vi "SVFA Unit Conversion (Colormap).vi"(0 "colormap":T9, 1 "desired scaling":T2 {"dB reference (0: no change)" format="%.2f"}, 2 "spectral density desired":T1(ring), 4 "spectrum info in":T3={"channel name"="", "description"="", "x-axis units"=0, "spectral info"={"spectrum type"=enum."Power [Magnitude^2]", "linear/dB"=enum."linear", "window"=0, "window size"=0, "FFT size"=0}, "engineering units"=0, "custom label"="", "dB reference [EU]"=0.0, "peak units"=enum."rms", "weighting filter"=0, "spectral density?"=FALSE, "unit label"="", "spectrum skewed?"=FALSE, "complimentary spectrum units"=enum."none"} {"x-axis units" items=["Time (s)"=0, "Frequency-CB (Hz)"=1, "Frequency-CPB (Hz)"=1248, "Frequency-Arbitrary (Hz)"=2357, "Quefrency (s)"=2, "Revolutions (rev)"=3, "Order"=4, "Speed (RPM)"=11, "Speed (rad/s)"=21, "Index"=65535]; "weighting filter" items=["Linear", "A-weighting", "B-weighting", "C-weighting", "ITU-R 468-4", "Dolby", "CCITT", "C-message", "Wb", "Wc", "Wd", "We", "Wf", "Wh", "Wj", "Wk", "Wm", "AES17 20 kHz lowpass", "AES17 40 kHz lowpass", "AES17 20 kHz highpass", "AES17 40 kHz highpass"]; "dB reference [EU]" format="%.2f"; "engineering units" items=["custom..."=0, "V"=1, "A"=21, "C"=30, "pC"=31, "s"=32, "-"=29, "Pa"=2, "N"=20, "g"=3, "m/s^2"=4, "m/s"=5, "m"=6, "mm/s"=12, "mm"=13, "micron/s"=14, "micron"=15, "in/s^2"=7, "in/s"=8, "in"=9, "mil/s"=10, "mil"=11, "rad/s^2"=16, "rad/s"=17, "rad"=18, "deg/s^2"=26, "deg/s"=27, "deg"=28, "RPM"=22, "cycle/s^2"=23, "Hz"=24, "cycle"=25, "strain"=19]; "spectral info"."window" items=["None "=0, "Hanning"=1, "Hamming"=2, "Blackman-Harris"=3, "Exact Blackman"=4, "Blackman"=5, "Flat Top"=6, "4 Term B-Harris "=7, "7 Term B-Harris"=8, "Low Sidelobe"=9, "Force - Exponential"=10, "Gaussian"=62]}, 5 "error in (no error)":errorcluster) -> (14 "converted colormap":T9, 15 "unit label":string, 18 "spectrum info out":T3={"channel name"="", "description"="", "x-axis units"=0, "spectral info"={"spectrum type"=enum."Power [Magnitude^2]", "linear/dB"=enum."linear", "window"=0, "window size"=0, "FFT size"=0}, "engineering units"=0, "custom label"="", "dB reference [EU]"=0.0, "peak units"=enum."rms", "weighting filter"=0, "spectral density?"=FALSE, "unit label"="", "spectrum skewed?"=FALSE, "complimentary spectrum units"=enum."none"} {"x-axis units" items=["Time (s)"=0, "Frequency-CB (Hz)"=1, "Frequency-CPB (Hz)"=1248, "Frequency-Arbitrary (Hz)"=2357, "Quefrency (s)"=2, "Revolutions (rev)"=3, "Order"=4, "Speed (RPM)"=11, "Speed (rad/s)"=21, "Index"=65535]; "weighting filter" items=["Linear", "A-weighting", "B-weighting", "C-weighting", "ITU-R 468-4", "Dolby", "CCITT", "C-message", "Wb", "Wc", "Wd", "We", "Wf", "Wh", "Wj", "Wk", "Wm", "AES17 20 kHz lowpass", "AES17 40 kHz lowpass", "AES17 20 kHz highpass", "AES17 40 kHz highpass"]; "dB reference [EU]" format="%.2f"; "engineering units" items=["custom..."=0, "V"=1, "A"=21, "C"=30, "pC"=31, "s"=32, "-"=29, "Pa"=2, "N"=20, "g"=3, "m/s^2"=4, "m/s"=5, "m"=6, "mm/s"=12, "mm"=13, "micron/s"=14, "micron"=15, "in/s^2"=7, "in/s"=8, "in"=9, "mil/s"=10, "mil"=11, "rad/s^2"=16, "rad/s"=17, "rad"=18, "deg/s^2"=26, "deg/s"=27, "deg"=28, "RPM"=22, "cycle/s^2"=23, "Hz"=24, "cycle"=25, "strain"=19]; "spectral info"."window" items=["None "=0, "Hanning"=1, "Hamming"=2, "Blackman-Harris"=3, "Exact Blackman"=4, "Blackman"=5, "Flat Top"=6, "4 Term B-Harris "=7, "7 Term B-Harris"=8, "Low Sidelobe"=9, "Force - Exponential"=10, "Gaussian"=62]}, 19 "error out":errorcluster)   [LabVIEW 2017]
doc: "Converts between dB/linear, magnitude/magnitude^2, rms/peak/peak-peak, spectrum/spectral density, and dB ref1/dB ref2. Wire data to the <B>spectrum</B> input to determine the polymorphic instance to use or manually select the instance."
uses:
  <vilib>/addons/_NISVFA/_Shared subVIs/Controls/svc_Spectrum Info.ctl
  <vilib>/addons/_NISVFA/_Shared subVIs/Controls/svc_X-Axis Units.ctl
  <vilib>/addons/_NISVFA/_Shared subVIs/Controls/svc_Spectrum Type.ctl
  <vilib>/addons/_NISVFA/_Shared subVIs/Controls/svc_Engineering Units Text Ring.ctl
  <vilib>/addons/_NISVFA/_Shared subVIs/Controls/svc_Weighting Filter Text Ring.ctl
  <vilib>/addons/_NISVFA/_Shared subVIs/Controls/svc_Complimentary Spectrum Units.ctl
  <vilib>/addons/_NISVFA/_Spectrum Processing/subVIs/svfa_Peak to RMS to Peak2Peak.vi
  <vilib>/addons/_NISVFA/_Spectrum Processing/subVIs/svfa_Mag to Mag2.vi
  <vilib>/addons/_NISVFA/_Spectrum Processing/subVIs/svfa_Linear to dB.vi
  <vilib>/addons/_NISVFA/_Spectrum Processing/subVIs/svfa_dBrefA to dBrefB.vi
  <vilib>/addons/_NISVFA/_Spectrum Processing/subVIs/svfa_Spectrum to Spectral Density.vi
  <vilib>/addons/_NISVFA/_Shared subVIs/Common/svc_Get Weighting Enum and Labels.vi
  <vilib>/addons/_NISVFA/_Shared subVIs/Common/svc_Unit Label Lexical Class.vi
  <vilib>/addons/_NISVFA/_Shared subVIs/Common/svc_Engineering Units to Unit Label.vi
  <vilib>/addons/_NISVFA/_Shared subVIs/Common/svc_Format Value (DBL).vi
  <vilib>/addons/_NISVFA/_Shared subVIs/Common/svc_Window Parameters.vi
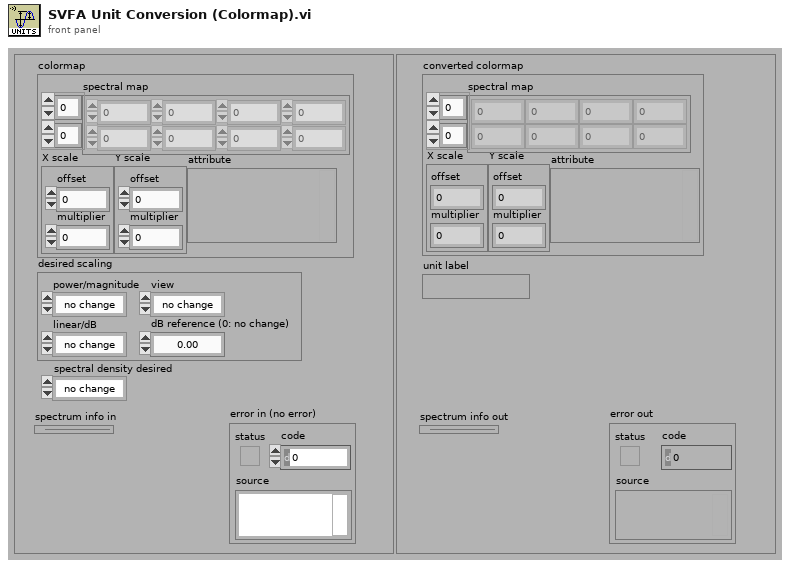
[diagram p1: front panel]
types:
  T1 = enum16{"no change", "spectrum", "spectral density"}
  T2 = cluster{"linear/dB":enum16{"no change", "linear", "dB"}, "dB reference (0: no change)":dbl, "power/magnitude":enum16{"no change", "power", "magnitude"}, "view":enum16{"no change", "rms", "peak", "peak-peak"}}
  T3 = typedef "svc_Spectrum Info.ctl" = cluster{"channel name":string, "description":string, "x-axis units":T4, "spectral info":cluster{"spectrum type":T5, "linear/dB":enum16{"linear", "dB"}, "window":u16, "window size":i32, "FFT size":i32}, "engineering units":T6, "custom label":string, "dB reference [EU]":dbl, "peak units":enum16{"rms", "peak", "peak-peak"}, "weighting filter":T7, "spectral density?":bool, "unit label":string, "spectrum skewed?":bool, "complimentary spectrum units":T8}
  T4 = typedef "svc_X-Axis Units.ctl" = u16
  T5 = typedef "svc_Spectrum Type.ctl" = enum16{"FFT Spectrum [complex]", "Amplitude [Magnitude]", "Power [Magnitude^2]", "Cross Spectrum [complex]", "Frequency Response [Complex]"}
  T6 = typedef "svc_Engineering Units Text Ring.ctl" = u16
  T7 = typedef "svc_Weighting Filter Text Ring.ctl" = u16
  T8 = typedef "svc_Complimentary Spectrum Units.ctl" = enum16{"none", "radians", "degrees", "cycles", "imaginary"}
  T9 = cluster{"spectral map":dbl[][], "X scale":cluster{"offset":dbl, "multiplier":dbl}, "Y scale":cluster{"offset":dbl, "multiplier":dbl}, "attribute":variant}
  T10 = enum16{"Frequency-Time", "Time-Frequency", "Order-Time", "Time-Order", "Frequency-RPM", "RPM-Frequency", "Order-RPM", "RPM-Order"}
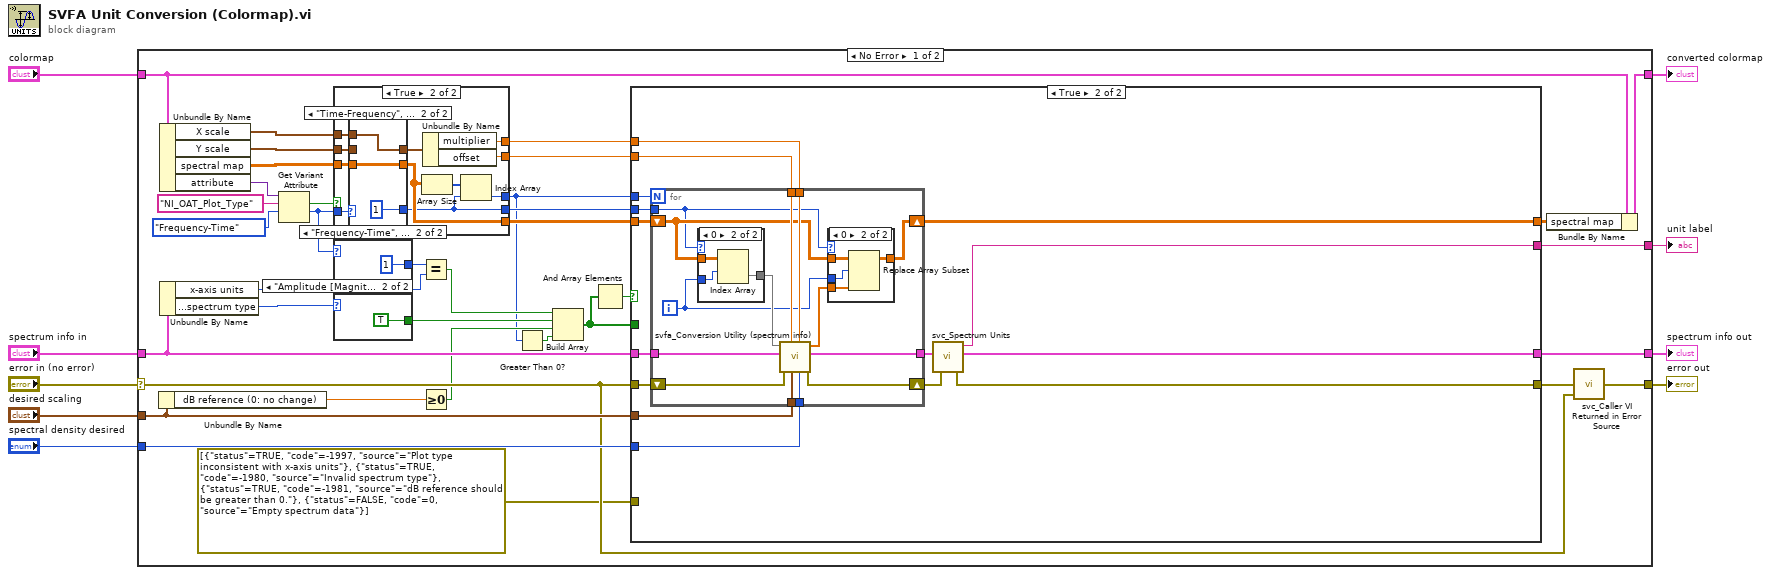
[diagram p0: block diagram]
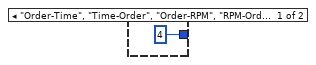
[diagram p2: hidden frame]
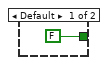
[diagram p3: hidden frame]
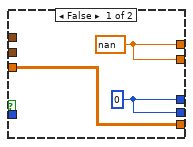
[diagram p4: hidden frame]
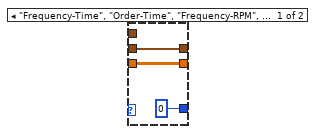
[diagram p5: hidden frame]
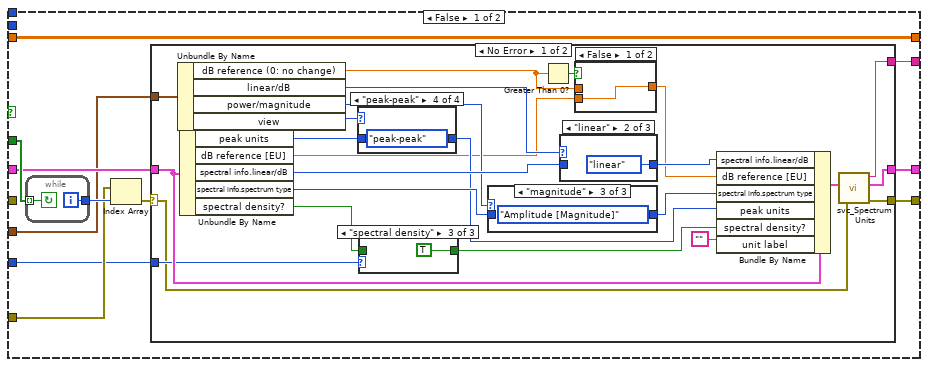
[diagram p6: hidden frame]
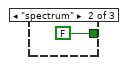
[diagram p8: hidden frame]
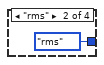
[diagram p10: hidden frame]
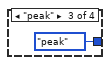
[diagram p11: hidden frame]
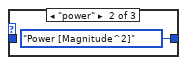
[diagram p13: hidden frame]
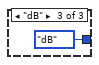
[diagram p16: hidden frame]
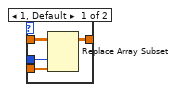
[diagram p18: hidden frame]
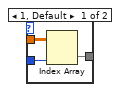
[diagram p19: hidden frame]
diagram:
  n1 = case shown="No Error" "error in (no error)" {
    selector: "error in (no error)" -> [w38 w168]
    tunnel: [w42 w168] -> w5
    tunnel: "desired scaling" -> [w41 _]
    tunnel: "spectrum info in" -> [w18 w167]
    tunnel: [w43 w167] -> w4
    tunnel: [w30 _] -> w3
    tunnel: "spectral density desired" -> [w40 _]
    tunnel: "colormap" -> [w29 w166]
    tunnel: [w24 w166] -> w2
    frame No Error {
      n2 = Unbundle By Name(w41) -> ("dB reference (0: no change)"=w39:dbl)
      n3 = Unbundle By Name(w29) -> ("X scale"=w35:cluster{"offset":dbl, "multiplier":dbl}, "Y scale"=w34:cluster{"offset":dbl, "multiplier":dbl}, "spectral map"=w25:dbl[][], "attribute"=w37:variant)
      n4 = Unbundle By Name(w18) -> ("x-axis units"=w20:T4, "spectral info.spectrum type"=w22:T5)
      n5 = Get Variant Attribute(Variant=w37, name="NI_OAT_Plot_Type", default value (empty Variant)=T10."Frequency-Time" ("plot type")) -> (found=w36:bool, value=w21:T10)  [unwired: 1 in, 2 out]
      n6 = case shown="True" w36 {
        tunnel: w25 -> [w51 w59]
        tunnel: [w51 w55] -> w31
        tunnel: w34 -> [_ w62]
        tunnel: w35 -> [_ w61]
        tunnel: w21 -> [_ w60]
        tunnel: [w49 w53] -> w13
        tunnel: [w50 w57] -> w27
        tunnel: [w50 w56] -> w26
        tunnel: [w49 w52] -> w23
        frame False {
          w49 = 0
          w50 = nan ("multiplier")
        }
        frame True {
          n7 = case shown="\"Time-Frequency\", \"Time-Order\", \"RPM-Frequency\", \"RPM-Order\"" w60 {
            tunnel: w59 -> [w64 w67]
            tunnel: w61 -> [_ w68]
            tunnel: w62 -> [w65 _]
            tunnel: [w64 w67] -> w55
            tunnel: [w65 w68] -> w58
            tunnel: [0 ("index") 1 ("index")] -> w52
            frame "Frequency-Time", "Order-Time", "Frequency-RPM", "Order-RPM", Default {
            }
            frame "Time-Frequency", "Time-Order", "RPM-Frequency", "RPM-Order" {
            }
          }
          n8 = Array Size(array=w55) -> (size(s)=w54:i32[])
          n9 = Unbundle By Name(w58) -> ("multiplier"=w57:dbl, "offset"=w56:dbl)
          n10 = Index Array(array=w54, index=w52) -> (element=w53:i32)
        }
      }
      n11 = case shown="\"Frequency-Time\", \"Time-Frequency\", \"Frequency-RPM\", \"RPM-Frequency\"" w21 {
        tunnel: [u16 4 ("x") u16 1 ("x")] -> w19
        frame "Order-Time", "Time-Order", "Order-RPM", "RPM-Order", Default {
        }
        frame "Frequency-Time", "Time-Frequency", "Frequency-RPM", "RPM-Frequency" {
        }
      }
      n12 = case shown="\"Amplitude [Magnitude]\", \"Power [Magnitude^2]\"" w22 {
        tunnel: [FALSE TRUE] -> w16
        frame Default {
        }
        frame "Amplitude [Magnitude]", "Power [Magnitude^2]" {
        }
      }
      n13 = Equal?(x=w19, y=w20) -> (x = y?=w17:bool)
      n14 = Greater Or Equal To 0?(x=w39) -> (x >= 0?=w15:bool)
      n15 = Greater Than 0?(x=w13) -> (x > 0?=w11:bool)
      n16 = Build Array(w17, w16, w15, w11) -> (w12:bool[])
      n17 = And Array Elements(Boolean array=w12) -> (logical AND=w14:bool)
      n18 = case shown="True" w14 {
        tunnel: w41 -> [w70 w136]
        tunnel: [w75 w135] -> w44
        tunnel: [w72 w134] -> w30
        tunnel: [w73 w133] -> w43
        tunnel: w18 -> [w74 w132]
        tunnel: w40 -> [w69 w131]
        tunnel: w27 -> [_ w130]
        tunnel: w26 -> [_ w129]
        tunnel: w31 -> [w79 w128]
        tunnel: w13 -> [_ w127]
        tunnel: [w79 w126] -> w28
        tunnel: w23 -> [_ w125]
        tunnel: w12 -> [w78 _]
        tunnel: errorcluster[] [{"status"=TRUE, "code"=-1997, "source"="Plot type inconsistent with x-axis units"}, {"status"=TRUE, "code"=-1980, "source"="Invalid spectrum type"}, {"status"=TRUE, "code"=-1981, "source"="dB reference should be greater than 0."}, {"status"=FALSE, "code"=0, "source"="Empty spectrum data"}] -> [w71 _]
        tunnel: w38 -> [_ w137]
        frame False {
          n19 = while {
            tunnel: w78 -> [w122] mode=indexing
            tunnel: [w121] -> w77
            i -> [w121]
            stop <- w122 continue-if-true
          }
          n20 = Index Array(array=w71, index=w77) -> (element=w76:errorcluster)
          n21 = case shown="No Error" w76 {
            selector: w76 -> [w86 w120]
            tunnel: [w85 w120] -> w75
            tunnel: w74 -> [w88 w119]
            tunnel: [w81 w119] -> w73
            tunnel: [w90 _] -> w72
            tunnel: w70 -> [w89 _]
            tunnel: w69 -> [w87 _]
            frame No Error {
              n22 = Unbundle By Name(w89) -> ("dB reference (0: no change)"=w99:dbl, "linear/dB"=w84:enum16{"no change", "linear", "dB"}, "power/magnitude"=w97:enum16{"no change", "power", "magnitude"}, "view"=w94:enum16{"no change", "rms", "peak", "peak-peak"})
              n23 = Unbundle By Name(w88) -> ("peak units"=w82:enum16{"rms", "peak", "peak-peak"}, "dB reference [EU]"=w83:dbl, "spectral info.linear/dB"=w102:enum16{"linear", "dB"}, "spectral info.spectrum type"=w96:T5, "spectral density?"=w92:bool)
              n24 = case shown="\"peak-peak\"" w94 {
                tunnel: w82 -> [w107 _ _ _]
                tunnel: [w107 enum16{"rms", "peak", "peak-peak"}."rms" ("peak units") enum16{"rms", "peak", "peak-peak"}."peak" ("peak units") enum16{"rms", "peak", "peak-peak"}."peak-peak" ("peak units")] -> w93
                frame "no change", Default {
                }
                frame "rms" {
                }
                frame "peak" {
                }
                frame "peak-peak" {
                }
              }
              n25 = case shown="\"spectral density\"" w87 {
                tunnel: w92 -> [w104 _ _]
                tunnel: [w104 FALSE ("spectral density?") TRUE ("spectral density?")] -> w91
                frame "no change", Default {
                }
                frame "spectrum" {
                }
                frame "spectral density" {
                }
              }
              n26 = case shown="\"magnitude\"" w97 {
                tunnel: w96 -> [w111 _ _]
                tunnel: [w111 svc_Spectrum_Type."Power [Magnitude^2]" ("spectrum type") svc_Spectrum_Type."Amplitude [Magnitude]" ("spectrum type")] -> w95
                frame "no change", Default {
                }
                frame "power" {
                }
                frame "magnitude" {
                }
              }
              n27 = Greater Than 0?(x=w99) -> (x > 0?=w100:bool)
              n28 = case shown="\"linear\"" w84 {
                tunnel: w102 -> [w116 _ _]
                tunnel: [w116 enum16{"linear", "dB"}."linear" ("linear/dB") enum16{"linear", "dB"}."dB" ("linear/dB")] -> w101
                frame "no change", Default {
                }
                frame "linear" {
                }
                frame "dB" {
                }
              }
              n29 = case shown="False" w100 {
                tunnel: w99 -> [_ w115]
                tunnel: [w114 w115] -> w98
                tunnel: w83 -> [w114 _]
                frame False {
                }
                frame True {
                }
              }
              n30 = Bundle By Name(cluster=w88, "spectral info.linear/dB"=w101, "dB reference [EU]"=w98, "spectral info.spectrum type"=w95, "peak units"=w93, "spectral density?"=w91, "unit label"="") -> (w80:T3)
              n31 = call <vilib>:"svc_Spectrum Units.vi"("error in (no error)"=w86, "spectrum info in"=w80) -> ("error out"=w85:errorcluster, "spectrum info out"=w81:T3, "unit label"=w90:string)  [unwired: 2 in, 1 out]
            }
            frame Error {
            }
          }
        }
        frame True {
          n32 = for {
            N: w127 -> [_]
            tunnel: w136 -> [w151]
            tunnel: w132 -> [w150]
            tunnel: [w148] -> w123
            tunnel: w131 -> [w147]
            tunnel: w130 -> [w146]
            tunnel: w129 -> [w145]
            shift-right: [w149] -> w124
            shift-left: w137 -> [w144]
            shift-right: [w140] -> w126
            shift-left: w128 -> [w142]
            tunnel: w125 -> [w138]
            i -> [w139]
            n33 = case shown="0" w138 {
              tunnel: w142 -> [w162 w165]
              tunnel: w139 -> [w161 w164]
              tunnel: [w160 w163] -> w143
              frame 1, Default {
                n34 = Index Array(array=w162, index (col)=w161) -> (element=w160:dbl[])  [unwired: 1 in]
              }
              frame 0 {
                n35 = Index Array(array=w165, index (row)=w164) -> (element=w163:dbl[])  [unwired: 1 in]
              }
            }
            n36 = call <vilib>:"svfa_Conversion Utility (spectrum info).vi"("spectral density desired"=w147, "dx"=w146, "desired scaling"=w151, "x0"=w145, "error in (no error)"=w144, "spectrum info in"=w150, "input signal"=w143) -> ("error out"=w149:errorcluster, "spectrum info out"=w148:T3, "converted signal"=w141:dbl[])  [unwired: 2 in]
            n37 = case shown="0" w138 {
              tunnel: w142 -> [w155 w159]
              tunnel: w141 -> [w154 w158]
              tunnel: w139 -> [w153 w157]
              tunnel: [w152 w156] -> w140
              frame 1, Default {
                n38 = Replace Array Subset(array=w155, new element=w154, index (col)=w153) -> (w152:dbl[][])  [unwired: 1 in]
              }
              frame 0 {
                n39 = Replace Array Subset(array=w159, new element=w158, index (row)=w157) -> (w156:dbl[][])  [unwired: 1 in]
              }
            }
          }
          n40 = call <vilib>:"svc_Spectrum Units.vi"("error in (no error)"=w124, "spectrum info in"=w123) -> ("error out"=w135:errorcluster, "spectrum info out"=w133:T3, "unit label"=w134:string)  [unwired: 2 in, 1 out]
        }
      }
      n41 = Bundle By Name(cluster=w29, "spectral map"=w28) -> (w24:T9)
      n42 = call <vilib>:"svc_Caller VI Returned in Error Source.vi"("warning input to caller"=w38, "error in (no error)"=w44) -> ("error out"=w42:errorcluster)  [unwired: 3 in]
    }
    frame Error {
    }
  }
  "error out" <- w5
  "converted colormap" <- w2
  "spectrum info out" <- w4
  "unit label" <- w3
